vi "OrientedDefense.vi"(0 "object in":refnum<class "DefendGoalTactic.lvclass">, 5 "error in (no error)":errorcluster) -> (14 "object out":refnum<class "DefendGoalTactic.lvclass">, 19 "error out":errorcluster)   [LabVIEW 2024, in "DefendGoalTactic.lvclass"]
uses:
  DefendGoalTactic.lvclass
  Game_class/Game.lvclass
  Robot_class/Robot.lvclass
  Game_class/Game.lvclass/Game.ctl
  Parameters_class/Parameters.lvclass/Parameters.ctl
  Game_class/Read FieldRef.vi
  Game_class/Read Parameters.lvclass.vi
  Parameters_class/Read GoalieInFrontGoal.vi
  Field_class/Field.lvclass
  Parameters_class/Parameters.lvclass
panel:
  in  "Robot":refnum<class "Robot.lvclass">
  in  "Game":refnum<class "Game.lvclass">
  in  "Y quina":dbl format="%#_13g"
  out "Orientação goleiro":dbl format="%#_13g"
  out "X goleiro":dbl format="%#_13g"
  out "Y golerio":dbl format="%#_13g"
  in  "Meio?":bool=TRUE
  in  "Orientação inimigo":dbl format="%#_13g"
  in  "Y bola":dbl format="%#_13g"
  in  "X bola":dbl format="%#_13g"
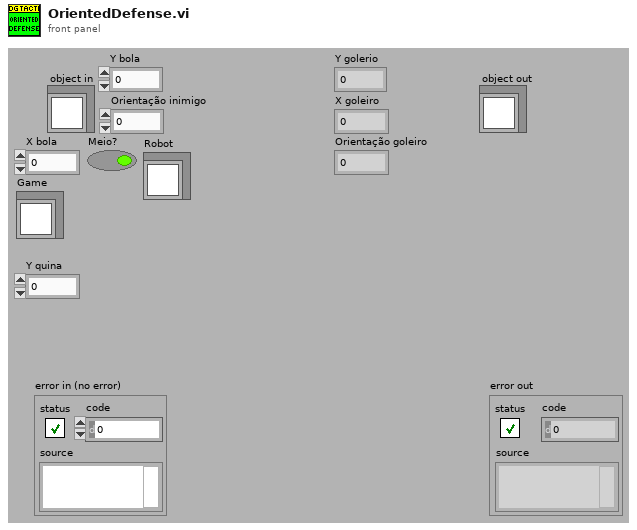
[diagram p1: front panel]
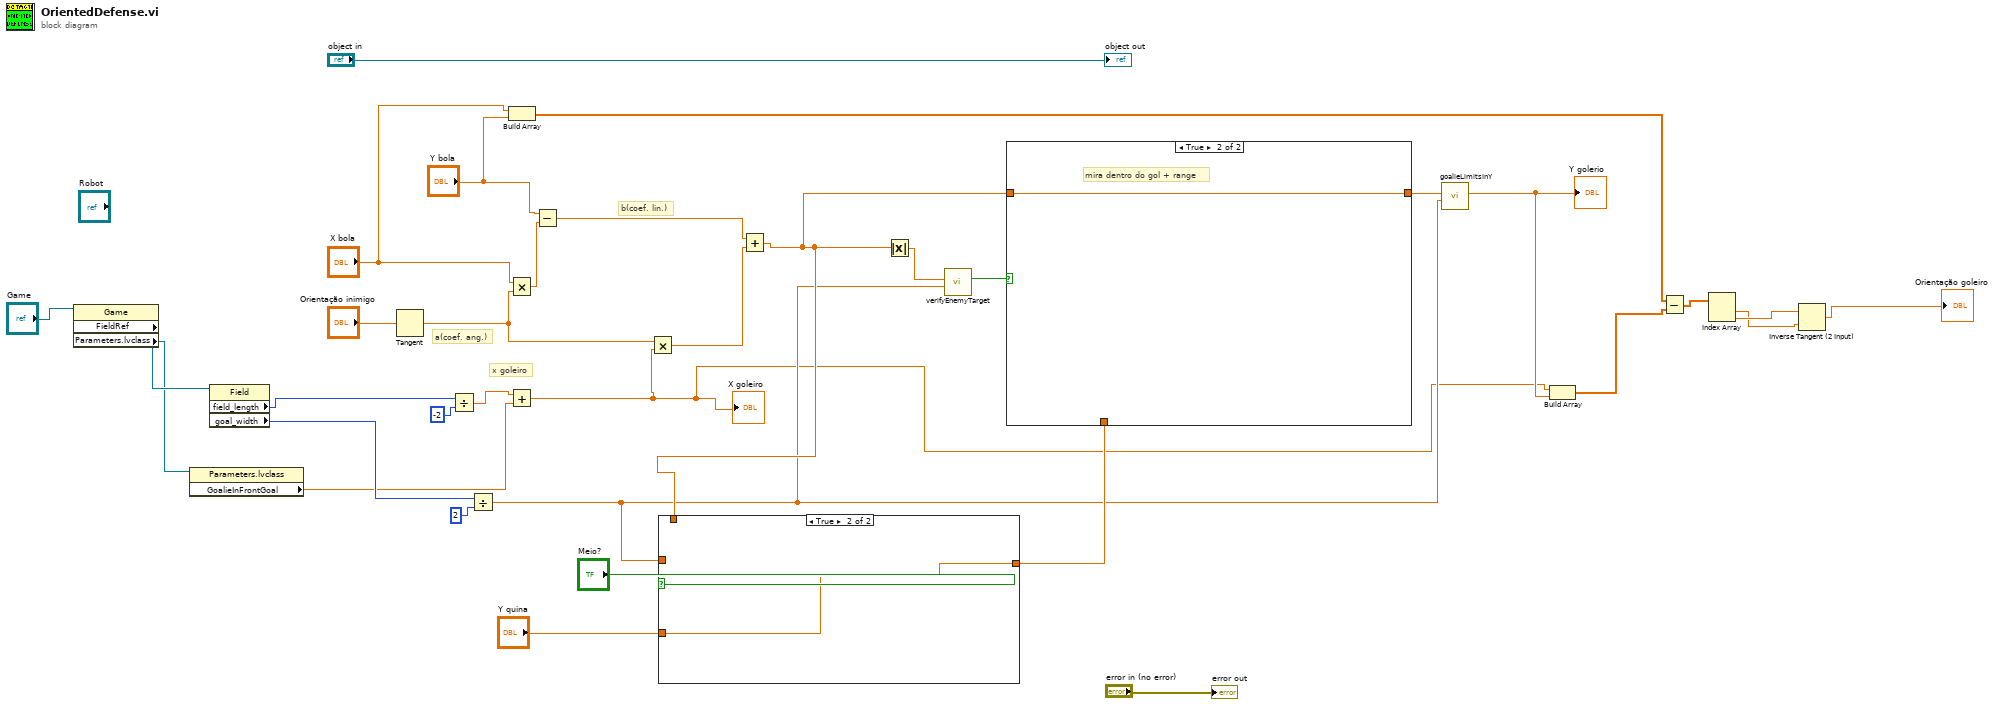
[diagram p0: block diagram]
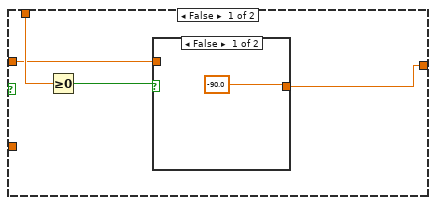
[diagram p2: hidden frame]
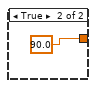
[diagram p3: hidden frame]
diagram:
  # "b(coef. lin.)"
  # "x goleiro"
  # "a(coef. ang.)"
  n1 = property class="Game"(reference="Game") -> ("FieldRef"=w4:refnum<class "Field.lvclass">, "Parameters.lvclass"=w3:refnum<class "Parameters.lvclass">)  [unwired: 1 in, 2 out]
  n2 = property class="Parameters.lvclass"(reference=w3) -> ("GoalieInFrontGoal"=w2:dbl)  [unwired: 1 in, 2 out]
  n3 = property class="Field"(reference=w4) -> ("field_length"=w6:i32, "goal_width"=w7:i32)  [unwired: 1 in, 2 out]
  n4 = Tangent(1:"Orientação inimigo") -> (0:w31:dbl)
  n5 = Divide(x=w6, y=-2) -> (x/y=w32:dbl)
  n6 = Divide(x=w7, y=2) -> (x/y=w10:dbl)
  n7 = Build Array("X bola", "Y bola") -> (w20:dbl[])
  n8 = Multiply(x="X bola", y=w31) -> (x*y=w34:dbl)
  n9 = Add(x=w32, y=w2) -> (x+y=w1:dbl)
  "X goleiro" <- w1
  n10 = Subtract(x="Y bola", y=w34) -> (x-y=w30:dbl)
  n11 = Multiply(x=w31, y=w1) -> (x*y=w29:dbl)
  n12 = Add(x=w30, y=w29) -> (x+y=w25:dbl)
  n13 = case shown="True" "Meio?" {
    tunnel: [w35 w41] -> w26
    tunnel: w25 -> [w38 _]
    tunnel: w10 -> [w36 _]
    tunnel: "Y quina" -> [_ w41]
    frame False {
      n14 = Greater Or Equal To 0?(x=w38) -> (x >= 0?=w37:bool)
      n15 = case shown="False" w37 {
        tunnel: w36 -> [_ _]
        tunnel: [-90.0 ("y") 90.0 ("y")] -> w35
        frame False {
        }
        frame True {
        }
      }
    }
    frame True {
    }
  }
  n16 = Absolute Value(x=w25) -> (abs(x)=w13:dbl)
  n17 = call "verifyEnemyTarget.vi"("GoalWidth/2"=w10, "EnemtyTargetInModlue"=w13) -> ("TargetInsideGoal"=w14:bool)  [unwired: 7 in, 2 out]
  n18 = case shown="True" w14 {
    tunnel: [w42 w43] -> w12
    tunnel: w25 -> [_ w43]
    tunnel: w26 -> [w42 _]
    frame False {
    }
    frame True {
      # "mira dentro do gol + range"
    }
  }
  n19 = call "goalieLimitsInY.vi"("Goal Width/2"=w10, "calculated Y"=w12) -> ("coerced Y"=w11:dbl)  [unwired: 7 in, 2 out]
  "Y golerio" <- w11
  n20 = Build Array(w1, w11) -> (w19:dbl[])
  n21 = Subtract(x=w20, y=w19) -> (x-y=w18:dbl[])
  n22 = Index Array(array=w18) -> (element #1=w16:dbl, element #2=w17:dbl)  [unwired: 2 in]
  n23 = Inverse Tangent (2 Input)(1:w16, 2:w17) -> (0:→"Orientação goleiro":dbl)
  "error out" <- "error in (no error)"
  "object out" <- "object in"
